vi "Save to csv_velocityMode.vi"() -> ()   [LabVIEW 2020]
uses:
  <vilib>/Utility/file.llb/Write Delimited Spreadsheet (string).vi
  <vilib>/Utility/file.llb/Write Delimited Spreadsheet (DBL).vi
panel:
  out "ID output velocity (rpm)":dbl[](array[numeric])
  in  "time (ms)":i32=5000
  in  "Save Path":path
  in  "Load data":bool
  in  "Save to csv":bool
  out "ID input velocity (rpm)":dbl[](array[numeric])
  out "time":dbl[](array[numeric])
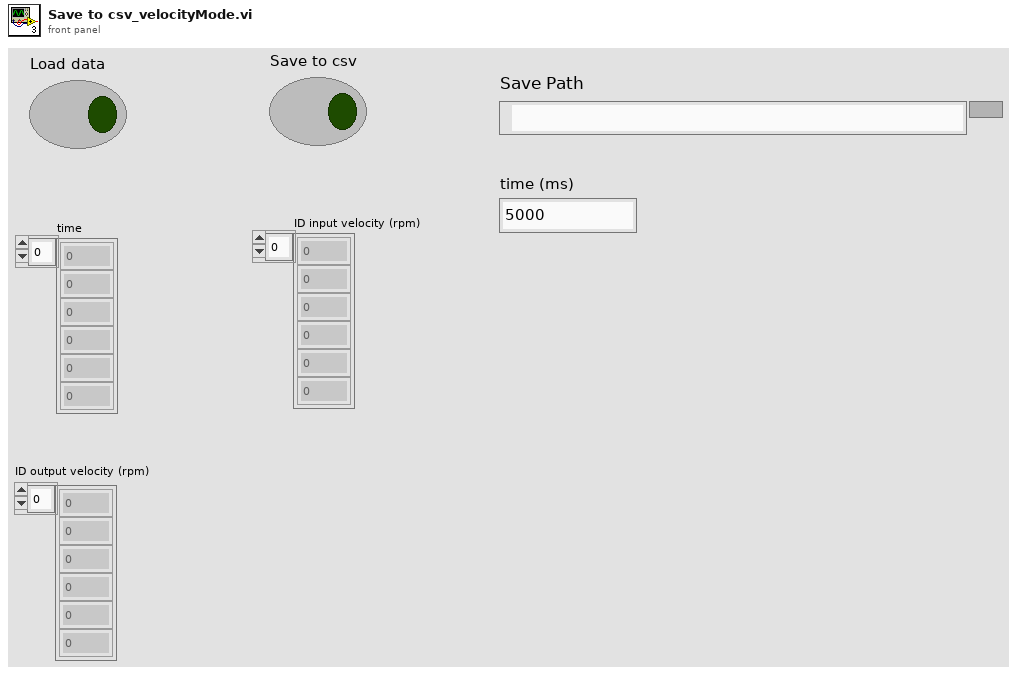
[diagram p1: front panel]
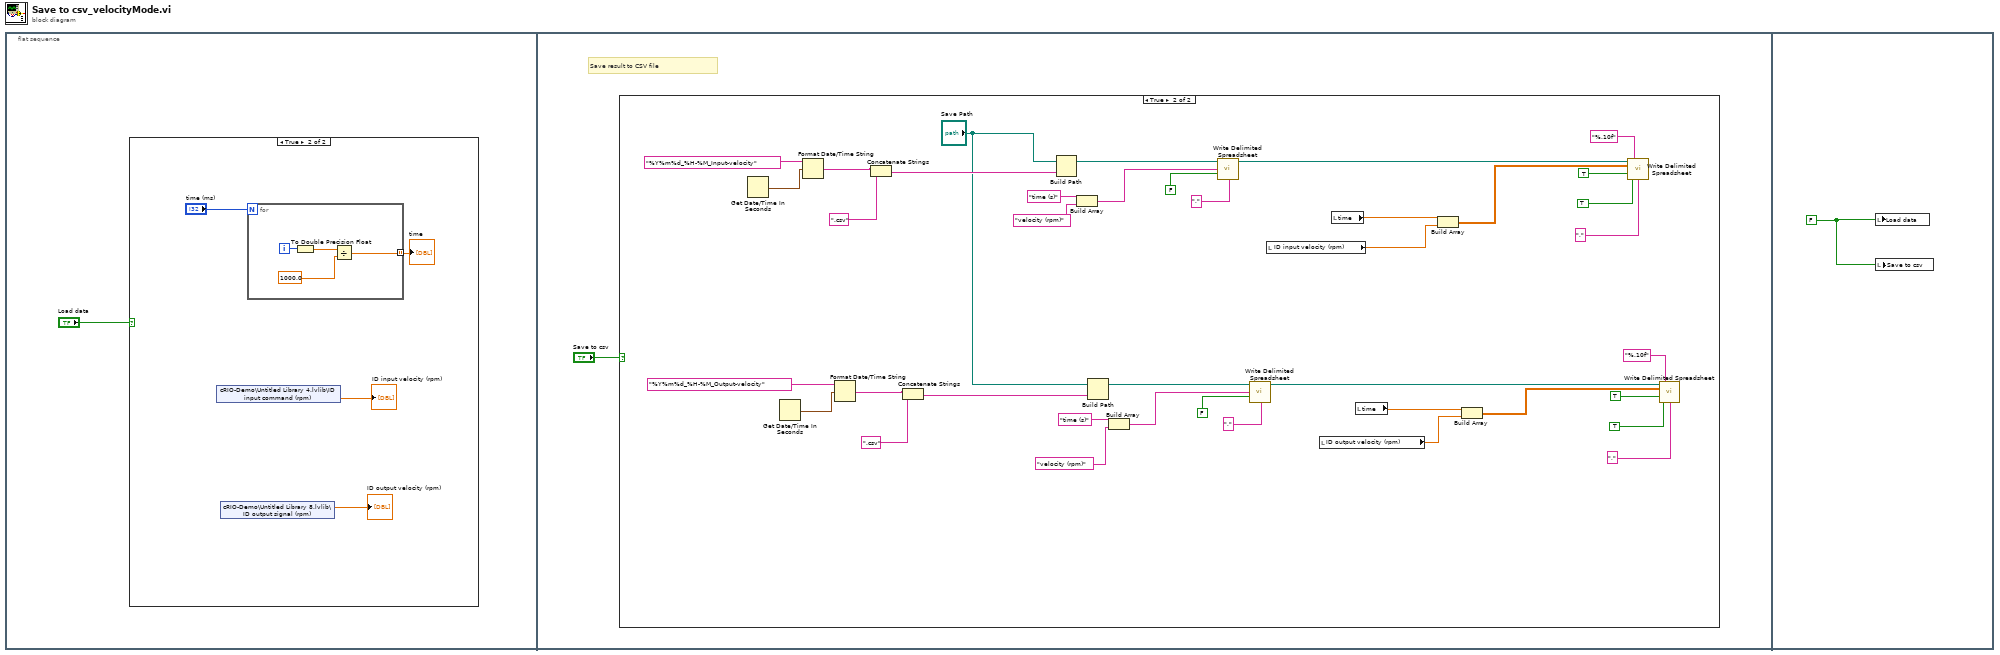
[diagram p0: block diagram]
diagram:
  n1 = flat-sequence {
    frame #0 {
      n2 = case shown="True" "Load data" {
        frame False {
        }
        frame True {
          n3 = shared-variable "cRIO-Demo\\Untitled Library 4.lvlib\\ID input command (rpm)"() -> (→"ID input velocity (rpm)":dbl[])  [unwired: 1 in, 1 out]
          n4 = shared-variable "cRIO-Demo\\Untitled Library 8.lvlib\\ID output signal (rpm)"() -> (→"ID output velocity (rpm)":dbl[])  [unwired: 1 in, 1 out]
          n5 = for {
            N: "time (ms)" -> [_]
            tunnel: [w6] -> w5 mode=indexing
            i -> [w9]
            n6 = To Double Precision Float(number=w9) -> (double precision float=w7:dbl)
            n7 = Divide(x=w7, y=1000.0) -> (x/y=w6:dbl)
          }
          "time" <- w5
        }
      }
    }
    frame #1 {
      # "Save result to CSV file"
      n8 = case shown="True" "Save to csv" {
        frame False {
        }
        frame True {
          n9 = Get Date/Time In Seconds() -> (seconds since 1Jan1904=w48:timestamp)
          n10 = Get Date/Time In Seconds() -> (seconds since 1Jan1904=w31:timestamp)
          n11 = Format Date/Time String(time format string (%c)="%Y%m%d_%H-%M_Input-velocity", seconds (now)=w48) -> (date/time string=w47:string)  [unwired: 1 in]
          n12 = Format Date/Time String(time format string (%c)="%Y%m%d_%H-%M_Output-velocity", seconds (now)=w31) -> (date/time string=w30:string)  [unwired: 1 in]
          n13 = Concatenate Strings(w47, ".csv") -> (w45:string)
          n14 = Concatenate Strings(w30, ".csv") -> (w28:string)
          n15 = Build Path(base path="Save Path", name or relative path=w45) -> (appended path=w44:path)
          n16 = Build Array("time (s)", "velocity (rpm)") -> (w35:string[])
          n17 = Build Path(base path="Save Path", name or relative path=w28) -> (appended path=w27:path)
          n18 = Build Array("time (s)", "velocity (rpm)") -> (w19:string[])
          n19 = call-poly <vilib>:"Write Delimited Spreadsheet.vi"("file path (dialog if empty)"=w44, "1D data"=w35, "append to file? (new file:F)"=FALSE, "delimiter (\\t)"=",") -> ("new file path (Not A Path if cancelled)"=w40:path)  [unwired: 10 in, 1 out]
          n20 = call-poly <vilib>:"Write Delimited Spreadsheet.vi"("file path (dialog if empty)"=w27, "1D data"=w19, "append to file? (new file:F)"=FALSE, "delimiter (\\t)"=",") -> ("new file path (Not A Path if cancelled)"=w23:path)  [unwired: 10 in, 1 out]
          n21 = local read "ID input velocity (rpm)"() -> (w15:dbl[])
          n22 = local read "ID output velocity (rpm)"() -> (w16:dbl[])
          n23 = local read "time"() -> (w33:dbl[])
          n24 = local read "time"() -> (w17:dbl[])
          n25 = Build Array(w33, w15) -> (w42:dbl[][])
          n26 = Build Array(w17, w16) -> (w25:dbl[][])
          n27 = call-poly <vilib>:"Write Delimited Spreadsheet.vi"("file path (dialog if empty)"=w40, "format (%.3f)"="%.10f", "2D data"=w42, "append to file? (new file:F)"=TRUE, "transpose? (no:F)"=TRUE, "delimiter (\\t)"=",") -> ()  [unwired: 8 in, 2 out]
          n28 = call-poly <vilib>:"Write Delimited Spreadsheet.vi"("file path (dialog if empty)"=w23, "format (%.3f)"="%.10f", "2D data"=w25, "append to file? (new file:F)"=TRUE, "transpose? (no:F)"=TRUE, "delimiter (\\t)"=",") -> ()  [unwired: 8 in, 2 out]
        }
      }
    }
    frame #2 {
      w50 = FALSE
      n29 = local write "Load data"(w50) -> ()
      n30 = local write "Save to csv"(w50) -> ()
    }
  }
